vi "UTIL_dynamic Error logger start v2_0_1.vi"(8 "error in (no error)":errorcluster, 10 "Error File Path":path=path "C:/Error Log.txt", 11 "Error.vi Path":path) -> (0 "error out":errorcluster, 3 "Error Ref out":refnum<vi>)   [LabVIEW 2015]
doc: "Util_dynamic Error logger start.vi\n\nThis vi is used to dynamically start the Error Q.vi. use it to cleanly launch error logger. \n\nCreated 2006 by:\n\nJ. Daren Suntych\nNational Analytics\n970-397-0764"
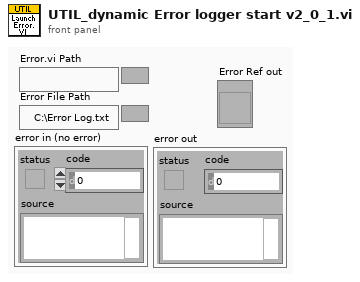
[diagram p1: front panel]
types:
  T1 = enum32{"Invalid", "Standard", "Closed", "Hidden", "Minimized", "Maximized"}
  T2 = enum32{"Bad", "Idle", "Run top level", "Running"}
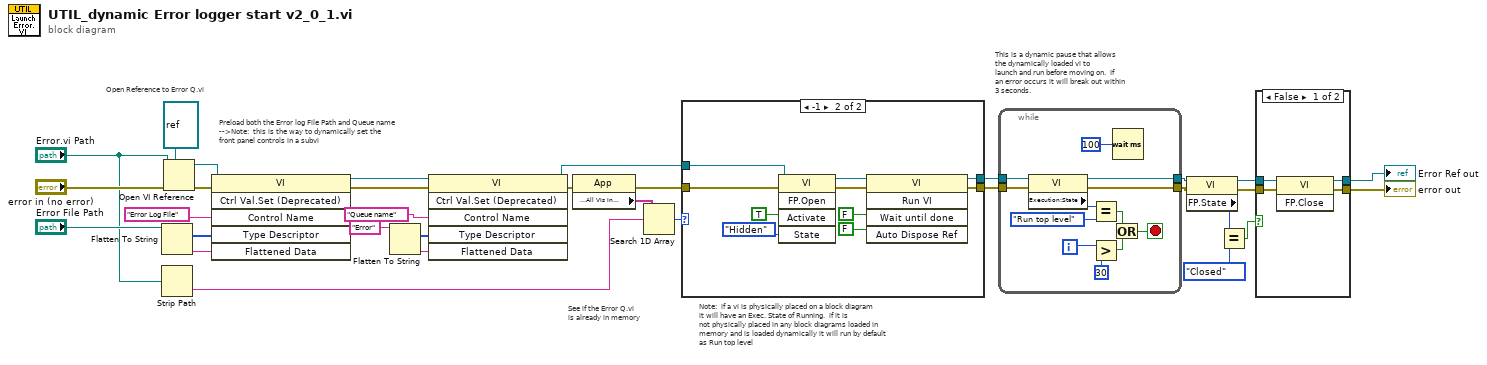
[diagram p0: block diagram]
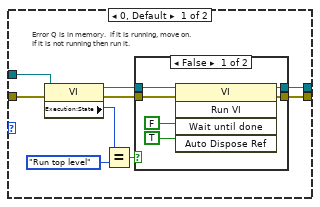
[diagram p3: hidden frame]
diagram:
  # "This is a dynamic pause that allows\nthe dynamically loaded vi to \nlaunch and run before moving on.  If \nan error occurs it will break out within\n3 seconds."
  # "Note:  if a vi is physically placed on a block diagram\nit will have an Exec. State of Running.  if it is\nnot physically placed in any block diagrams loaded in\nmemory and is loaded dynamically it will run by default\nas Run top level"
  # "Preload both the Error log File Path and Queue name\n-->Note:  this is the way to dynamically set the \nfront panel controls in a subvi"
  # "Open Reference to Error Q.vi"
  # "See if the Error Q.vi\nis already in memory"
  n1 = Flatten To String(anything="Error File Path") -> (data string=w28:string, type string=w29:i16[])  [unwired: 1 in, 3 out]
  n2 = Strip Path(path="Error.vi Path") -> (name=w10:string)  [unwired: 1 out]
  n3 = Open VI Reference(type specifier VI Refnum (for type only)=refnum<vi> refnum, vi path="Error.vi Path", error in (no error)="error in (no error)") -> (vi reference=w32:refnum<vi>, error out=w31:errorcluster)  [unwired: 3 out]
  n4 = invoke class="VI" method="Ctrl Val.Set (Deprecated)"(reference=w32, error in=w31, "Control Name"="Error Log File", "Type Descriptor"=w29, "Flattened Data"=w28) -> (reference out=w13:refnum<vi>, error out=w16:errorcluster)  [unwired: 1 in, 4 out]
  n5 = Flatten To String(anything="Error" ("Control Name")) -> (data string=w19:string, type string=w18:i16[])  [unwired: 1 in, 3 out]
  n6 = invoke class="VI" method="Ctrl Val.Set (Deprecated)"(reference=w13, error in=w16, "Control Name"="Queue name", "Type Descriptor"=w18, "Flattened Data"=w19) -> (reference out=w14:refnum<vi>, error out=w15:errorcluster)  [unwired: 1 in, 4 out]
  n7 = property class="App"(error in=w15) -> (error out=w20:errorcluster, "Application:All VIs In Memory"=w25:string[])  [unwired: 1 in, 1 out]
  n8 = Search 1D Array(1D array=w25, element=w10) -> (index of element=w24:i32)  [unwired: 1 out]
  n9 = case shown="-1" w24 {
    tunnel: w20 -> [w39 w59]
    tunnel: [w41 w51] -> w23
    tunnel: [w40 w53] -> w22
    tunnel: w14 -> [w33 w50]
    frame 0, Default {
      # "Error Q is in memory.  if it is running, move on.\nIf it is not running then run it."
      n10 = property class="VI"(reference=w33, error in=w39) -> (reference out=w37:refnum<vi>, error out=w38:errorcluster, "Execution:State"=w36:T2)
      n11 = Equal?(x=w36, y=T2."Run top level") -> (x = y?=w34:bool)
      n12 = case shown="False" w34 {
        tunnel: [w46 w48] -> w41
        tunnel: [w45 w49] -> w40
        tunnel: w38 -> [w44 w48]
        tunnel: w37 -> [w43 w49]
        frame False {
          n13 = invoke class="VI" method="Run VI"(reference=w43, error in=w44, "Wait until done"=FALSE, "Auto Dispose Ref"=TRUE ("Wait until done")) -> (reference out=w45:refnum<vi>, error out=w46:errorcluster)  [unwired: 1 in, 3 out]
        }
        frame True {
        }
      }
    }
    frame -1 {
      n14 = invoke class="VI" method="FP.Open"(reference=w50, error in=w59, "Activate"=TRUE, "State"=T1."Hidden") -> (reference out=w54:refnum<vi>, error out=w52:errorcluster)  [unwired: 1 in, 3 out]
      n15 = invoke class="VI" method="Run VI"(reference=w54, error in=w52, "Wait until done"=FALSE, "Auto Dispose Ref"=FALSE ("Wait until done")) -> (reference out=w53:refnum<vi>, error out=w51:errorcluster)  [unwired: 1 in, 3 out]
    }
  }
  n16 = while {
    tunnel: w22 -> [w71]
    tunnel: w23 -> [w70]
    tunnel: [w62] -> w8
    tunnel: [w60] -> w9
    i -> [w67]
    stop <- w63 stop-if-true
    n17 = property class="VI"(reference=w71, error in=w70) -> (reference out=w60:refnum<vi>, error out=w62:errorcluster, "Execution:State"=w69:T2)
    n18 = Equal?(x=w69, y=T2."Run top level" ("Execution:State")) -> (x = y?=w65:bool)
    n19 = Greater?(x=w67, y=30) -> (0:w64:bool)
    n20 = Or(x=w65, y=w64) -> (x .or. y?=w63:bool)
    n21 = Wait (ms)(milliseconds to wait=u32 100) -> ()  [unwired: 1 out]
  }
  n22 = property class="VI"(reference=w9, error in=w8) -> (reference out=w4:refnum<vi>, error out=w3:errorcluster, "FP.State"=w7:T1)
  n23 = Equal?(x=w7, y=T1."Closed" ("Front Panel Window:State")) -> (x = y?=w5:bool)
  n24 = case shown="False" w5 {
    tunnel: [w72 w77] -> w1
    tunnel: w4 -> [w75 w77]
    tunnel: [w73 w76] -> w2
    tunnel: w3 -> [w74 w76]
    frame False {
      n25 = invoke class="VI" method="FP.Close"(reference=w75, error in=w74) -> (reference out=w72:refnum<vi>, error out=w73:errorcluster)  [unwired: 1 in, 1 out]
    }
    frame True {
    }
  }
  "error out" <- w2
  "Error Ref out" <- w1
